vi "IO参数设置.vi"(8 "布尔文本.文本":string, 9 "section (optional)":string, 10 "监测项描述":string) -> (1 "簇2输出":T2, 2 "增加？":bool, 3 "簇1输出":T1)   [LabVIEW 2016, in "环境动力监测库.lvlib"]
uses:
  <vilib>/Utility/miscctls.llb/LVPointTypeDef.ctl
  <vilib>/Utility/config.llb/NI_LVConfig.lvlib
panel:
  in  "传感器型号:":enum16{"PLC", "ZLAN"}(ring)
  in  "簇1输入":T1
  in  "簇2输入":T2
  in  "返回":bool
  in  "增加":bool
  in  "信息接收人:":cluster{"管理员":bool, "普通用户":bool}
  in  "告警解除内容:":string
  in  "告警解除方式:":T3
  in  "告警电话内容:":string
  in  "告警短信内容:":string
  in  "告警抓拍设置:":enum16{"无"}(ring)
  in  "告警时段选择:":T4(ring)
  in  "告警发送方式:":T3
  in  "重复告警时间\n(s):":i16
  in  "预警保持时间\n(s):":i16
  in  "模板选择:":T5(ring)
  in  "告警参数:":enum32{"禁用告警", "闭合告警", "断开告警"}(radio)
  in  "端口:":T6(ring)
  in  "监测项描述:":string
  # "基本设置"
  # "如:红外XX"
  # "传感器选择"
  # "端口选择"
  # "参数设置"
  # "告警方式选择"
  # "告警设置"
  # "数值范围: 0~9999"
  # "数值范围: 0~9999"
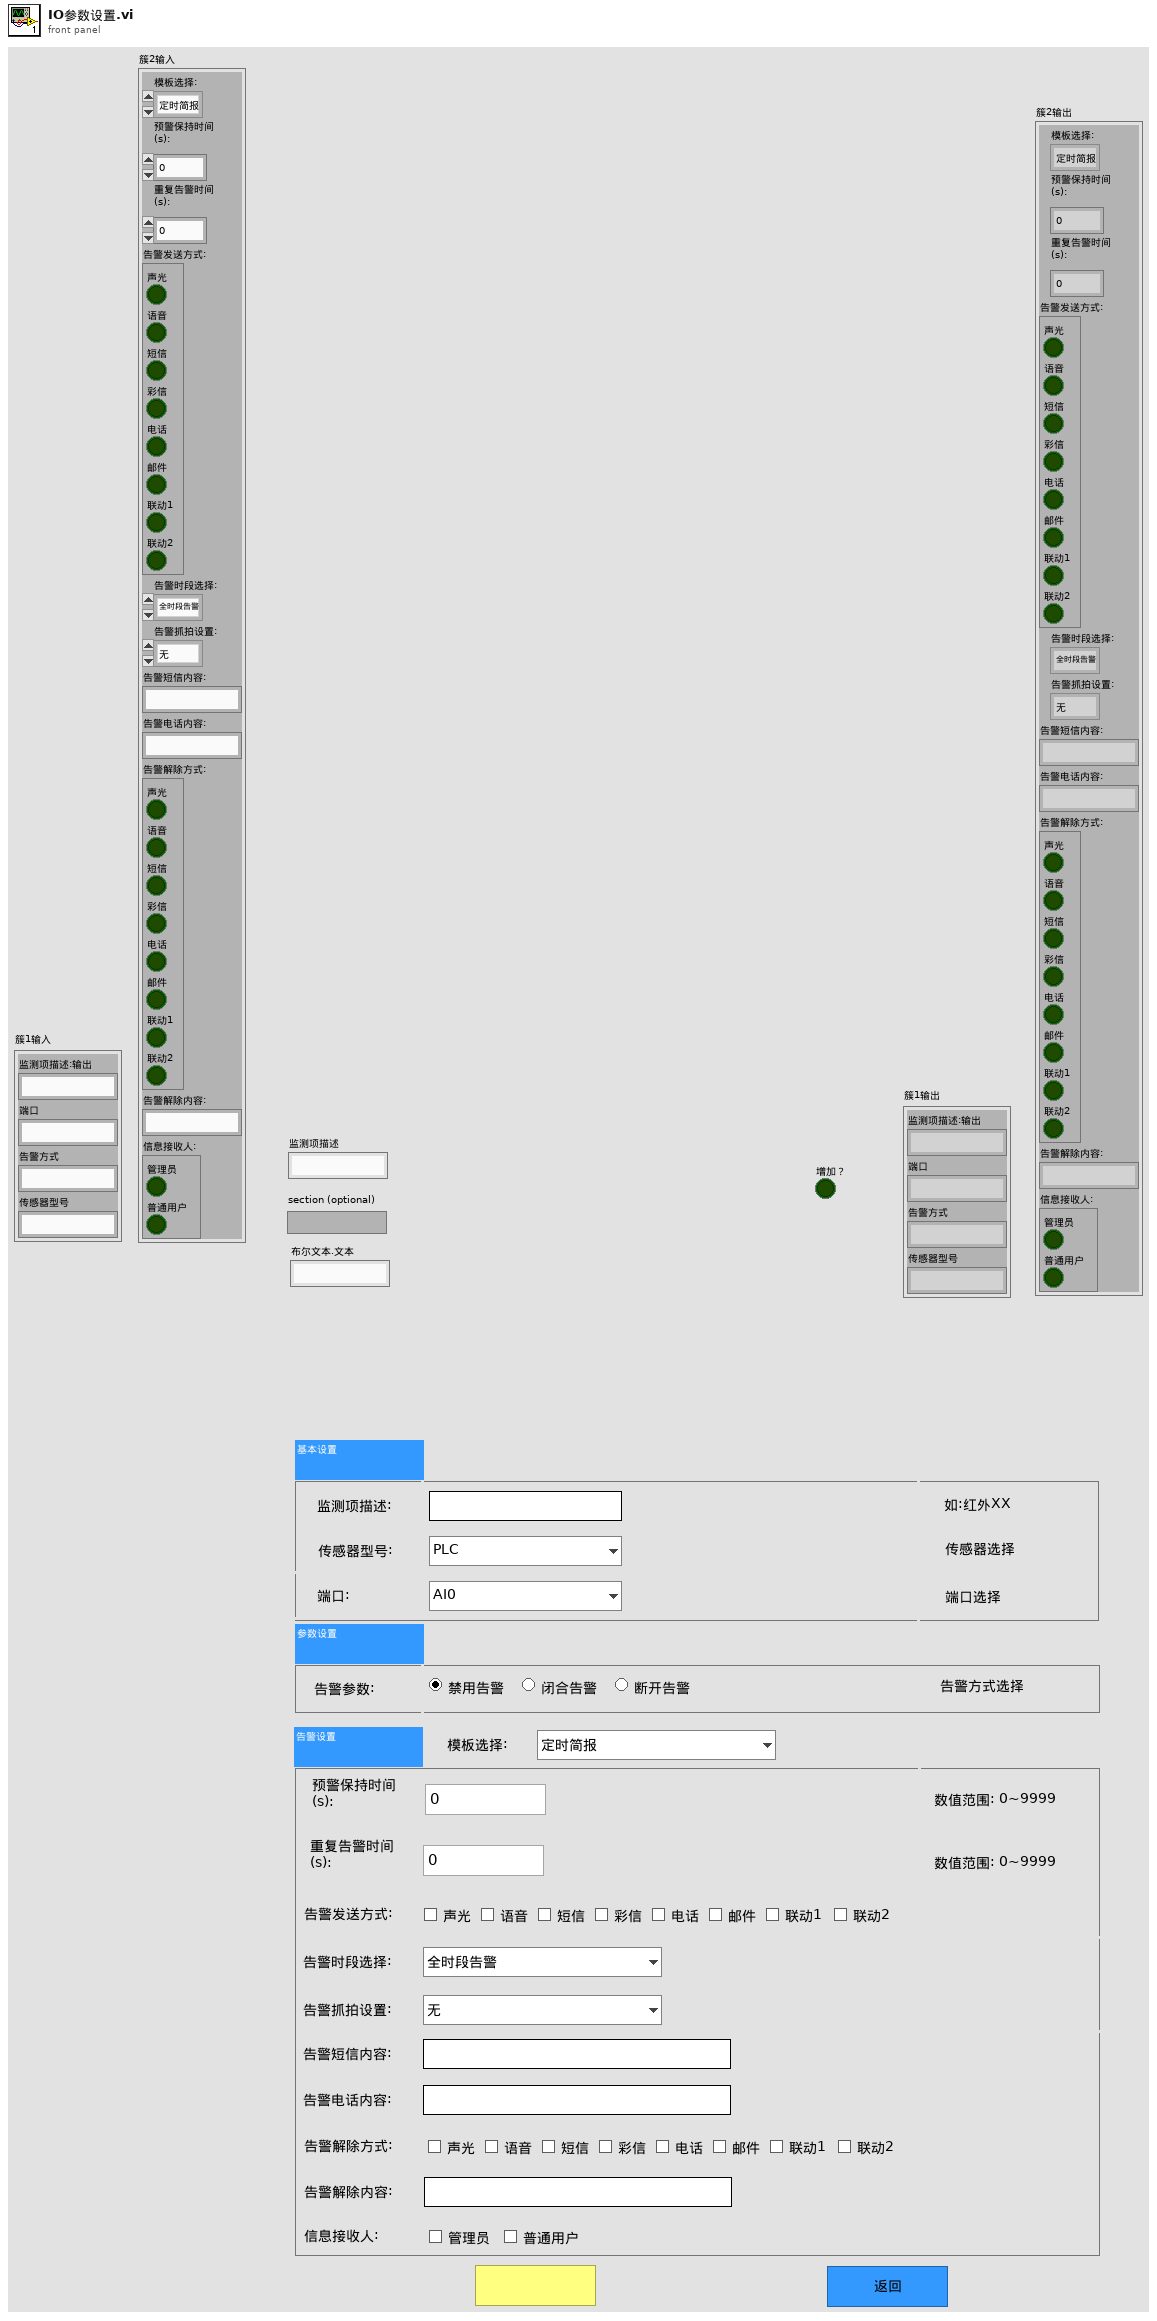
[diagram p1: front panel]
types:
  T1 = cluster{"监测项描述:输出":string, "端口":string, "告警方式":string, "传感器型号":string}
  T2 = cluster{"模板选择:":enum16{"定时简报", "无(不告警)", "通用声光告警", "通用语言告警", "通用短信告警", "通用电话告警", "通用邮件告警", "通用声光+语音+短信告警", "通用声光+短信+电话告警", "通用多方式告警", "通用全方式告警", "自动按类型", "非告警时段", "自定义"}, "预警保持时间\n(s):":i16, "重复告警时间\n(s):":i16, "告警发送方式:":cluster{"声光":bool, "语音":bool, "短信":bool, "彩信":bool, "电话":bool, "邮件":bool, "联动1":bool, "联动2":bool}, "告警时段选择:":enum16{"全时段告警", "工作日告警", "周六周日告警", "非告警时段", "自定义"}, "告警抓拍设置:":enum16{"无"}, "告警短信内容:":string, "告警电话内容:":string, "告警解除方式:":cluster{"声光":bool, "语音":bool, "短信":bool, "彩信":bool, "电话":bool, "邮件":bool, "联动1":bool, "联动2":bool}, "告警解除内容:":string, "信息接收人:":cluster{"管理员":bool, "普通用户":bool}}
  T3 = cluster{"声光":bool, "语音":bool, "短信":bool, "彩信":bool, "电话":bool, "邮件":bool, "联动1":bool, "联动2":bool}
  T4 = enum16{"全时段告警", "工作日告警", "周六周日告警", "非告警时段", "自定义"}
  T5 = enum16{"定时简报", "无(不告警)", "通用声光告警", "通用语言告警", "通用短信告警", "通用电话告警", "通用邮件告警", "通用声光+语音+短信告警", "通用声光+短信+电话告警", "通用多方式告警", "通用全方式告警", "自动按类型", "非告警时段", "自定义"}
  T6 = enum16{"AI0", "AI1", "AI2", "AI3", "AI4", "DI0", "DI1", "DI2", "DI3", "DI4", "X0", "X1", "X2", "X3", "X4", "X5", "X6", "X7", "X8", "X9"}
  T7 = typedef "LVPointTypeDef.ctl" = cluster{"Horizontal":i16, "Vertical":i16}
  T8 = typedef "NI_LVConfig.lvlib/Config Data RefNum.ctl" = refnum<k1>
  T9 = cluster{"监测项描述:":string, "端口:":enum16{"AI0", "AI1", "AI2", "AI3", "AI4", "DI0", "DI1", "DI2", "DI3", "DI4", "X0", "X1", "X2", "X3", "X4", "X5", "X6", "X7", "X8", "X9"}, "告警参数:":enum32{"禁用告警", "闭合告警", "断开告警"}, "传感器型号:":enum16{"PLC", "ZLAN"}}
  T10 = cluster{"漏水监测配置":cluster{"监测项描述:输出":string, "端口:":enum16{"AI0", "AI1", "AI2", "AI3", "AI4", "DI0", "DI1", "DI2", "DI3", "DI4", "X0", "X1", "X2", "X3", "X4", "X5", "X6", "X7", "X8", "X9"}, "告警参数:":enum32{"禁用告警", "闭合告警", "断开告警"}, "传感器型号:":enum16{"PLC", "ZLAN"}}, "门禁开关监测配置":cluster{"监测项描述:输出":string, "端口:":enum16{"AI0", "AI1", "AI2", "AI3", "AI4", "DI0", "DI1", "DI2", "DI3", "DI4", "X0", "X1", "X2", "X3", "X4", "X5", "X6", "X7", "X8", "X9"}, "告警参数:":enum32{"禁用告警", "闭合告警", "断开告警"}, "传感器型号:":enum16{"PLC", "ZLAN"}}, "温湿度监测配置":cluster{"监测项描述:输出":string, "端口:":enum16{"AI0", "AI1", "AI2", "AI3", "AI4", "DI0", "DI1", "DI2", "DI3", "DI4", "X0", "X1", "X2", "X3", "X4", "X5", "X6", "X7", "X8", "X9"}, "告警参数:":enum32{"禁用告警", "闭合告警", "断开告警"}, "传感器型号:":enum16{"PLC", "ZLAN"}}, "烟雾监测配置":cluster{"监测项描述:输出":string, "端口:":enum16{"AI0", "AI1", "AI2", "AI3", "AI4", "DI0", "DI1", "DI2", "DI3", "DI4", "X0", "X1", "X2", "X3", "X4", "X5", "X6", "X7", "X8", "X9"}, "告警参数:":enum32{"禁用告警", "闭合告警", "断开告警"}, "传感器型号:":enum16{"PLC", "ZLAN"}}}
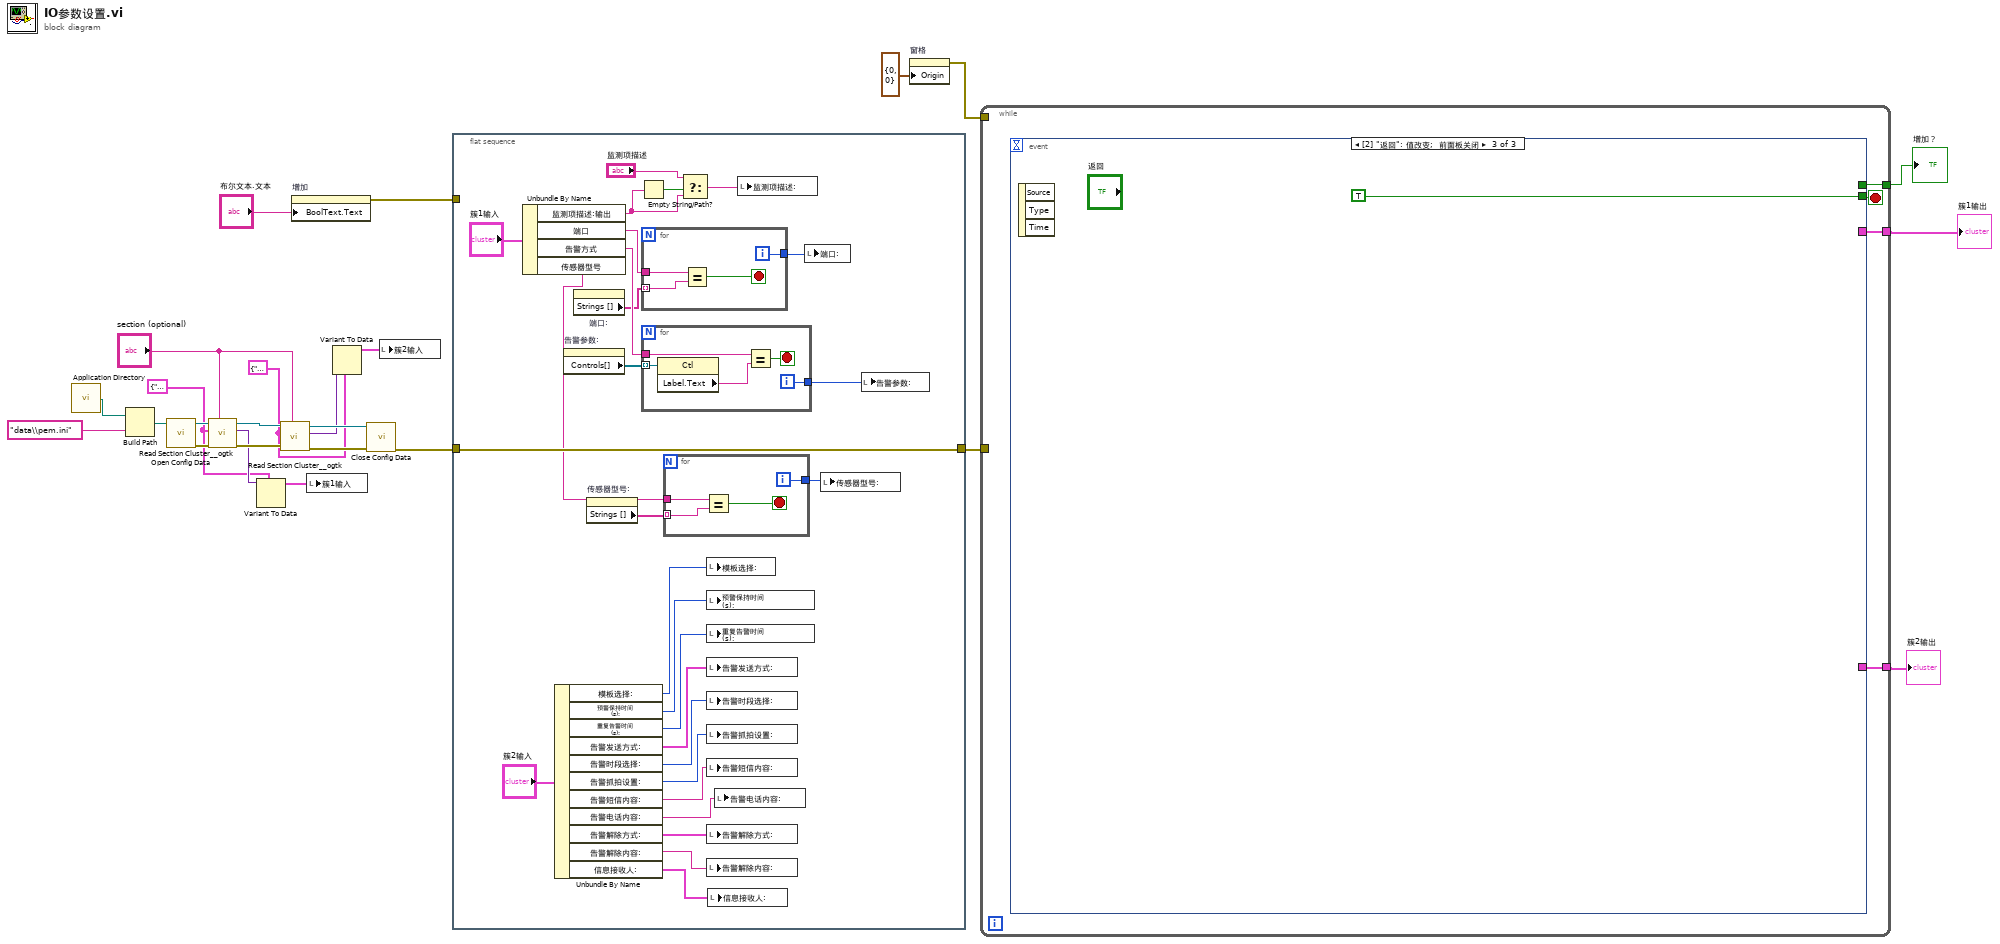
[diagram p0: block diagram]
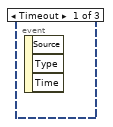
[diagram p2: hidden frame]
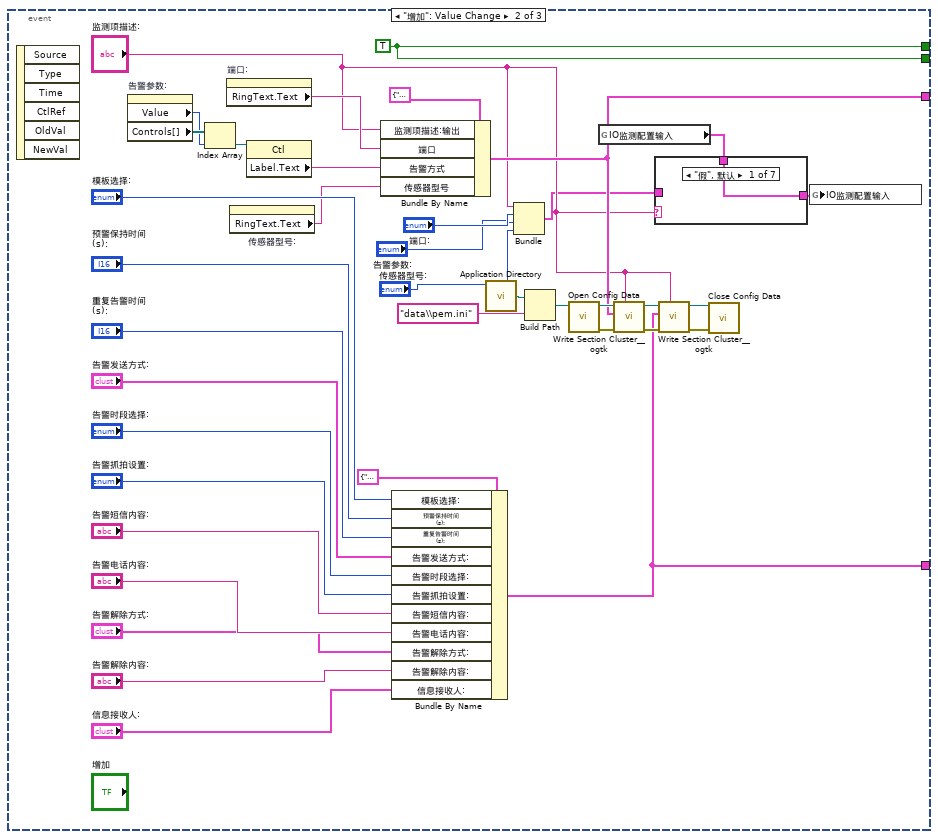
[diagram p3: hidden frame]
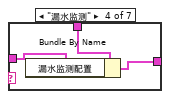
[diagram p6: hidden frame]
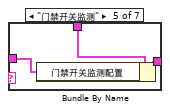
[diagram p7: hidden frame]
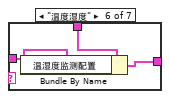
[diagram p8: hidden frame]
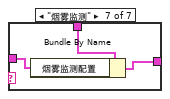
[diagram p9: hidden frame]
diagram:
  w1 = T2 {"模板选择:"=enum."定时简报", "预警保持时间\n(s):"=0, "重复告警时间\n(s):"=0, "告警发送方式:"={"声光"=FALSE, "语音"=FALSE, "短信"=FALSE, "彩信"=FALSE, "电话"=FALSE, "邮件"=FALSE, "联动1"=FALSE, "联动2"=FALSE}, "告警时段选择:"=enum."全时段告警", "告警抓拍设置:"=enum."无", "告警短信内容:"="", "告警电话内容:"="", "告警解除方式:"={"声光"=FALSE, "语音"=FALSE, "短信"=FALSE, "彩信"=FALSE, "电话"=FALSE, "邮件"=FALSE, "联动1"=FALSE, "联动2"=FALSE}, "告警解除内容:"="", "信息接收人:"={"管理员"=FALSE, "普通用户"=FALSE}} ("数据")
  w2 = T1 {"监测项描述:输出"="", "端口"="", "告警方式"="", "传感器型号"=""} ("簇1输入")
  n1 = call <vilib>:"Application Directory.vi"() -> ("Application Directory"=w18:path)
  n2 = Build Path(base path=w18, name or relative path="data\\pem.ini" ("名称或相对路径")) -> (appended path=w19:path)
  n3 = call <vilib>:"Open Config Data.vi"("configuration file path"=w19) -> ("error out"=w20:errorcluster, "refnum"=w22:T8)  [unwired: 8 in, 1 out]
  n4 = call <userlib>:"Read Section Cluster__ogtk.vi"("section (optional)"="section (optional)", "error in (no error)"=w20, "Section Formatted Cluster Type"=w2, "refnum"=w22) -> ("error out"=w15:errorcluster, "Section Formatted Cluster"=w12:variant, "dup refnum"=w21:T8)  [unwired: 3 in, 2 out]
  n5 = Variant To Data(type=w2, Variant=w12) -> (data=w3:T1)  [unwired: 1 in, 1 out]
  n6 = call <userlib>:"Read Section Cluster__ogtk.vi"("section (optional)"="section (optional)", "error in (no error)"=w15, "Section Formatted Cluster Type"=w1, "refnum"=w21) -> ("error out"=w14:errorcluster, "Section Formatted Cluster"=w11:variant, "dup refnum"=w16:T8)  [unwired: 3 in, 2 out]
  n7 = property on="增加" class="Bool"("BoolText.Text"="布尔文本.文本") -> (error out=w6:errorcluster)  [unwired: 2 in, 1 out]
  n8 = local write "簇1输入"(w3) -> ()
  n9 = Variant To Data(type=w1, Variant=w11) -> (data=w10:T2)  [unwired: 1 in, 1 out]
  n10 = call <vilib>:"Close Config Data.vi"("error in (no error)"=w14, "refnum"=w16) -> ("error out"=w9:errorcluster)  [unwired: 8 in, 1 out]
  n11 = local write "簇2输入"(w10) -> ()
  n12 = flat-sequence {
    tunnel: w9 -> [w33]
    tunnel: [w33] -> w8
    tunnel: w6 -> [_]
    frame #0 {
      n13 = Unbundle By Name("簇1输入") -> ("监测项描述:输出"=w30:string, "端口"=w35:string, "告警方式"=w38:string, "传感器型号"=w27:string)
      n14 = Unbundle By Name("簇2输入") -> ("模板选择:"=w50:T5, "预警保持时间\n(s):"=w49:i16, "重复告警时间\n(s):"=w48:i16, "告警发送方式:"=w47:T3, "告警时段选择:"=w46:T4, "告警抓拍设置:"=w45:enum16{"无"}, "告警短信内容:"=w44:string, "告警电话内容:"=w43:string, "告警解除方式:"=w42:T3, "告警解除内容:"=w41:string, "信息接收人:"=w40:cluster{"管理员":bool, "普通用户":bool})
      n15 = property on="告警参数:" class="RadioBtnsControl (严格)"() -> ("Controls[]"=w39:refnum<vi>[])  [unwired: 2 in, 2 out]
      n16 = property on="端口:" class="Enum (严格)"() -> ("Strings []"=w36:string[])  [unwired: 2 in, 2 out]
      n17 = property on="传感器型号:" class="Enum (严格)"() -> ("Strings []"=w28:string[])  [unwired: 2 in, 2 out]
      n18 = Empty String/Path?(string/path=w30) -> (empty?=w32:bool)
      n19 = for {
        tunnel: w35 -> [w60]
        tunnel: [w58] -> w34
        tunnel: w36 -> [w57] mode=indexing
        i -> [w58]
        stop <- w59 stop-if-true
        n20 = Equal?(x=w60, y=w57) -> (x = y?=w59:bool)
      }
      n21 = for {
        tunnel: w39 -> [w65] mode=indexing
        tunnel: w38 -> [w63]
        tunnel: [w61] -> w37
        i -> [w61]
        stop <- w62 stop-if-true
        n22 = property class="Ctl"(reference=w65) -> ("Label.Text"=w64:string)  [unwired: 1 in, 2 out]
        n23 = Equal?(x=w63, y=w64) -> (x = y?=w62:bool)
      }
      n24 = for {
        tunnel: w27 -> [w56]
        tunnel: [w54] -> w26
        tunnel: w28 -> [w53] mode=indexing
        i -> [w54]
        stop <- w55 stop-if-true
        n25 = Equal?(x=w56, y=w53) -> (x = y?=w55:bool)
      }
      n26 = Select(t="监测项描述", s=w32, f=w30) -> (s? t:f=w29:string)
      n27 = local write "模板选择:"(w50) -> ()
      n28 = local write "预警保持时间\n(s):"(w49) -> ()
      n29 = local write "重复告警时间\n(s):"(w48) -> ()
      n30 = local write "告警发送方式:"(w47) -> ()
      n31 = local write "告警时段选择:"(w46) -> ()
      n32 = local write "告警抓拍设置:"(w45) -> ()
      n33 = local write "告警短信内容:"(w44) -> ()
      n34 = local write "告警解除方式:"(w42) -> ()
      n35 = local write "告警解除内容:"(w41) -> ()
      n36 = local write "信息接收人:"(w40) -> ()
      n37 = local write "告警电话内容:"(w43) -> ()
      n38 = local write "监测项描述:"(w29) -> ()
      n39 = local write "端口:"(w34) -> ()
      n40 = local write "传感器型号:"(w26) -> ()
      n41 = local write "告警参数:"(w37) -> ()
    }
  }
  n42 = property on="窗格" class="Pane"("Origin"=T7 {"Horizontal"=0, "Vertical"=0} ("原点")) -> (error out=w23:errorcluster)  [unwired: 2 in, 1 out]
  n43 = while {
    tunnel: [w69] -> w4
    tunnel: [w67] -> w25
    tunnel: w23 -> [_]
    tunnel: [w66] -> w5
    tunnel: w8 -> [_]
    stop <- w68 stop-if-true
    n44 = event shown="[2] \"返回\": 值改变;  前面板关闭" {
      selector: _ -> [_ _ _]
      dyn-events: _ -> [_ _ _]
      timeout: _ -> [_ _ _]
      tunnel: [_ w107 TRUE] -> w68
      tunnel: [_ w75 _] -> w69
      tunnel: [_ w107 _] -> w67
      tunnel: [_ w81 _] -> w66
      event Timeout {
        n45 = event-data() -> ()  [unwired: 1 in, 3 out]
      }
      event "增加": Value Change {
        w107 = TRUE
        n46 = event-data() -> ()  [unwired: 1 in, 6 out]
        n47 = property on="告警参数:" class="RadioBtnsControl (严格)"() -> ("Value"=w105:enum32{"禁用告警", "闭合告警", "断开告警"}, "Controls[]"=w106:refnum<vi>[])  [unwired: 2 in, 2 out]
        n48 = Index Array(array=w106, index=w105) -> (element=w104:refnum<vi>)
        n49 = property on="端口:" class="Enum (严格)"() -> ("RingText.Text"=w103:string)  [unwired: 2 in, 2 out]
        n50 = property on="传感器型号:" class="Enum (严格)"() -> ("RingText.Text"=w78:string)  [unwired: 2 in, 2 out]
        n51 = property class="Ctl"(reference=w104) -> ("Label.Text"=w102:string)  [unwired: 1 in, 2 out]
        n52 = Bundle By Name(cluster=T1 {"监测项描述:输出"="", "端口"="", "告警方式"="", "传感器型号"=""} ("簇1输出"), "监测项描述:输出"="监测项描述:", "端口"=w103, "告警方式"=w102, "传感器型号"=w78) -> (w75:T1)
        n53 = Bundle By Name(cluster=T2 {"模板选择:"=enum."定时简报", "预警保持时间\n(s):"=0, "重复告警时间\n(s):"=0, "告警发送方式:"={"声光"=FALSE, "语音"=FALSE, "短信"=FALSE, "彩信"=FALSE, "电话"=FALSE, "邮件"=FALSE, "联动1"=FALSE, "联动2"=FALSE}, "告警时段选择:"=enum."全时段告警", "告警抓拍设置:"=enum."无", "告警短信内容:"="", "告警电话内容:"="", "告警解除方式:"={"声光"=FALSE, "语音"=FALSE, "短信"=FALSE, "彩信"=FALSE, "电话"=FALSE, "邮件"=FALSE, "联动1"=FALSE, "联动2"=FALSE}, "告警解除内容:"="", "信息接收人:"={"管理员"=FALSE, "普通用户"=FALSE}} ("簇2输出"), "模板选择:"="模板选择:", "预警保持时间\n(s):"="预警保持时间\n(s):", "重复告警时间\n(s):"="重复告警时间\n(s):", "告警发送方式:"="告警发送方式:", "告警时段选择:"="告警时段选择:", "告警抓拍设置:"="告警抓拍设置:", "告警短信内容:"="告警短信内容:", "告警电话内容:"="告警电话内容:", "告警解除方式:"="告警解除方式:", "告警解除内容:"="告警解除内容:", "信息接收人:"="信息接收人:") -> (w81:T2)
        n54 = call <vilib>:"Application Directory.vi"() -> ("Application Directory"=w87:path)
        n55 = Bundle("监测项描述:"="监测项描述:", "端口:"="端口:", "告警参数:"="告警参数:", "传感器型号:"="传感器型号:") -> (w70:T9)  [unwired: 1 in]
        n56 = Build Path(base path=w87, name or relative path="data\\pem.ini" ("名称或相对路径")) -> (appended path=w88:path)
        n57 = call <vilib>:"Open Config Data.vi"("configuration file path"=w88) -> ("error out"=w89:errorcluster, "refnum"=w90:T8)  [unwired: 8 in, 1 out]
        n58 = global read "内部交互全局变量.vi" "IO监测配置输入"() -> (w76:T10)
        n59 = call <userlib>:"Write Section Cluster__ogtk.vi"("section (optional)"="监测项描述:", "error in (no error)"=w89, "Section Formatted Cluster"=w75, "refnum"=w90) -> ("error out"=w84:errorcluster, "dup refnum"=w85:T8)  [unwired: 6 in]
        n60 = case shown="\"假\", 默认" "监测项描述:" {
          tunnel: w76 -> [w108 w109 w110 w113 w116 w119 w122]
          tunnel: [w108 w109 w110 w112 w115 w118 w121] -> w77
          tunnel: w70 -> [_ _ _ w111 w114 w117 w120]
          frame "假", Default {
          }
          frame "市电监测" {
          }
          frame "空调监测" {
          }
          frame "漏水监测" {
            n61 = Bundle By Name(cluster=w113, "漏水监测配置"=w111) -> (w112:T10)
          }
          frame "门禁开关监测" {
            n62 = Bundle By Name(cluster=w116, "门禁开关监测配置"=w114) -> (w115:T10)
          }
          frame "温度湿度" {
            n63 = Bundle By Name(cluster=w119, "温湿度监测配置"=w117) -> (w118:T10)
          }
          frame "烟雾监测" {
            n64 = Bundle By Name(cluster=w122, "烟雾监测配置"=w120) -> (w121:T10)
          }
        }
        n65 = call <userlib>:"Write Section Cluster__ogtk.vi"("section (optional)"="监测项描述:", "error in (no error)"=w84, "Section Formatted Cluster"=w81, "refnum"=w85) -> ("error out"=w82:errorcluster, "dup refnum"=w83:T8)  [unwired: 6 in]
        n66 = call <vilib>:"Close Config Data.vi"("error in (no error)"=w82, "refnum"=w83) -> ()  [unwired: 8 in, 2 out]
        n67 = global write "内部交互全局变量.vi" "IO监测配置输入"(w77) -> ()
      }
      event "返回": Value Change; Panel Close {
        n68 = event-data() -> ()  [unwired: 1 in, 3 out]
      }
    }
  }
  "增加？" <- w25
  "簇1输出" <- w4
  "簇2输出" <- w5
